vi "Update Cursor.vi"(8 "error in (no error)":errorcluster, 10 "Cursor":T1, 11 "Keypad in":refnum<class "Keypad.lvclass">) -> (0 "error out":errorcluster, 3 "Keypad out":refnum<class "Keypad.lvclass">)   [LabVIEW 2020, in "Keypad.lvlib" / "Keypad.lvclass"]
uses:
  Keypad.lvclass
  Type Def - Cursor Display.ctl
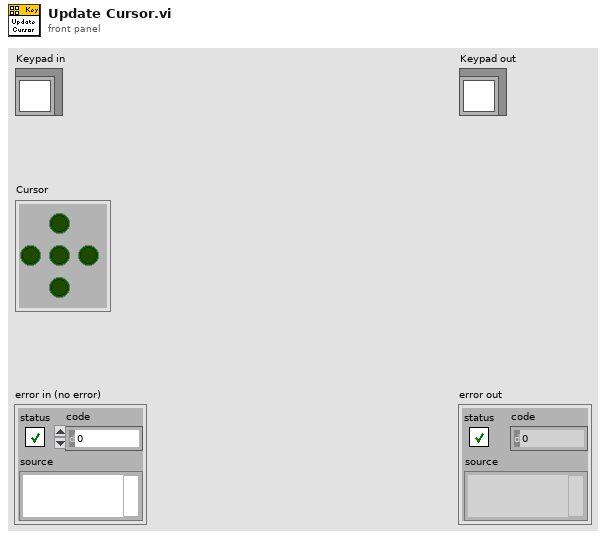
[diagram p1: front panel]
types:
  T1 = typedef "Type Def - Cursor Display.ctl" = cluster{"Up":bool, "Left":bool, "Ctr":bool, "Right":bool, "Down":bool}
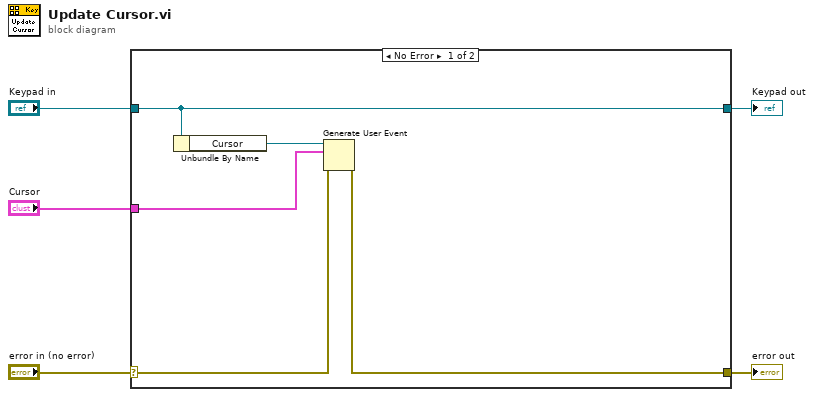
[diagram p0: block diagram]
diagram:
  n1 = case shown="No Error" "error in (no error)" {
    selector: "error in (no error)" -> [w8 w12]
    tunnel: [w7 w12] -> w4
    tunnel: [w10 w11] -> w2
    tunnel: "Keypad in" -> [w10 w11]
    tunnel: "Cursor" -> [w6 _]
    frame No Error {
      n2 = Unbundle By Name(w10) -> ("Cursor"=w9:refnum<user-event>)
      n3 = Generate User Event(user event=w9, event data cluster=w6, error in=w8) -> (error out=w7:errorcluster)  [unwired: 1 in, 1 out]
    }
    frame Error {
    }
  }
  "error out" <- w4
  "Keypad out" <- w2
